vi "Check for Flow Alarm.vi"(0 "Test Table":string[][](array[string]), 1 "Current Step ID":i32) -> ()   [LabVIEW 2012]
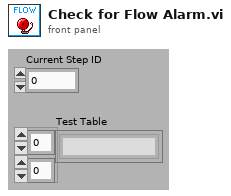
[diagram p1: front panel]
types:
  T1 = enum16{"Init", "Add Alarm Limits", "Update Flow Limit", "Check for Alarm", "Clear Alarms"}
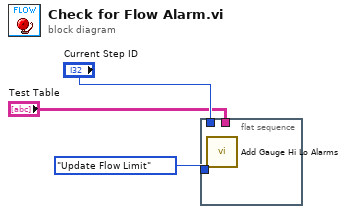
[diagram p0: block diagram]
diagram:
  n1 = flat-sequence {
    tunnel: T1."Update Flow Limit" ("Action") -> [w4]
    tunnel: "Test Table" -> [_]
    tunnel: "Current Step ID" -> [_]
    frame #0 {
      n2 = call "Add Gauge Hi Lo Alarms.vi"("Action"=w4) -> ()  [unwired: 10 in]
    }
  }
